vi "ProdaNG.Error.GetLastMsg.vi"(8 "error in":errorcluster, 11 "dbHandleIn":i32) -> (0 "error out":errorcluster, 2 "Last Error Message":string)   [LabVIEW 2016]
doc: "This function returns the text of the last ORACLE error for a defined context. This function can only be used with a valid Handle.\nParameter:\nhandle is an Integer, that is returned by the function Login() when a new connection is created.\nReturn Value:\nLast ORACLE error message\nIn case that a handle is invalid, an empty string is returned."
uses:
  prodllNG.dll
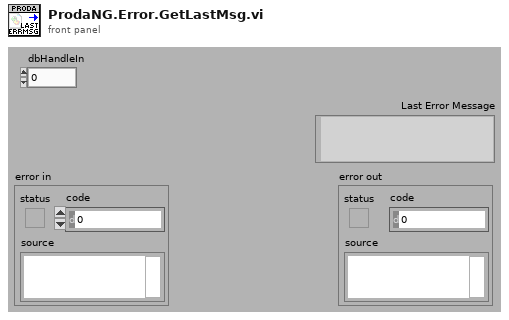
[diagram p1: front panel]
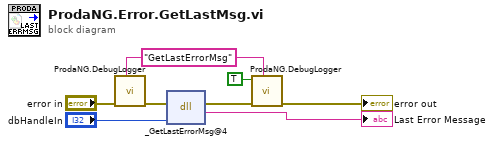
[diagram p0: block diagram]
diagram:
  w1 = "GetLastErrorMsg" ("cmd")
  n1 = call "ProdaNG.DebugLogger.vi"("cmd"=w1, "error in (no error)"="error in") -> ("error out"=w5:errorcluster)  [unwired: 9 in]
  n2 = dll-call lib="C:/LabviewSoftware/OP50-master/sources/Database/ProdaNG/prodllNG.dll" fn="_GetLastErrorMsg@4" ("ProDll.dll:Login")(error in=w5, "dbHandle"="dbHandleIn") -> (error out=w3:errorcluster, "return type"=→"Last Error Message":string)  [unwired: 3 in, 1 out]
  n3 = call "ProdaNG.DebugLogger.vi"("cmd"=w1, "error in (no error)"=w3, "done? (F)"=TRUE) -> ("error out"=→"error out":errorcluster)  [unwired: 8 in]
